vi "Send PING.vi"(8 "error in (no error)":errorcluster caption="entrée d'erreur (pas d'erreur)", 9 "timeout":i32=50, 10 "Frame Send":i32=10, 11 "@IP":string="192.168.0.100") -> (0 "error out":errorcluster caption="sortie d'erreur", 2 "Result/Request":bool[](array[boolean]), 3 "Result":bool)   [LabVIEW 2020, in "Library Commun.lvlib"]
uses:
  Library Commun.lvlib
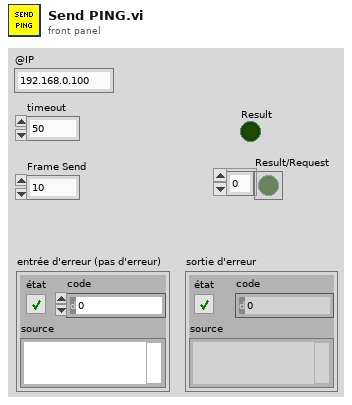
[diagram p1: front panel]
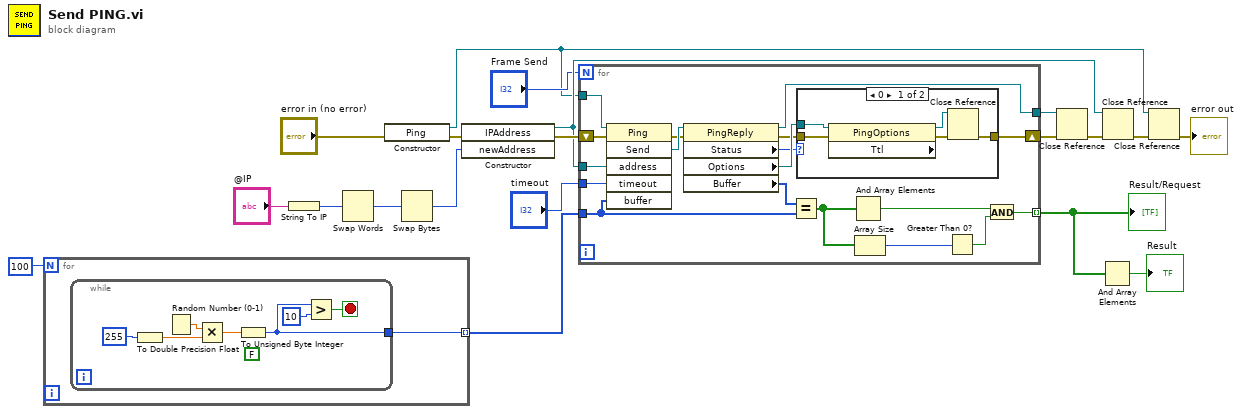
[diagram p0: block diagram]
diagram:
  n1 = for {
    N: 100 -> [_]
    tunnel: [w21] -> w9 mode=indexing
    n2 = while {
      tunnel: [w24] -> w21
      stop <- w22 stop-if-true
      (unwired) FALSE
      n3 = To Double Precision Float(number=u8 255 ("nombre")) -> (double precision float=w26:dbl)
      n4 = Random Number (0-1)() -> (number: 0 to 1=w27:dbl)
      n5 = Multiply(x=w27, y=w26) -> (x*y=w25:dbl)
      n6 = To Unsigned Byte Integer(number=w25) -> (unsigned 8bit integer=w24:u8)
      n7 = Greater?(x=w24, y=u8 10) -> (0:w22:bool)
    }
  }
  n8 = String To IP(1:"@IP") -> (0:w18:u32)
  n9 = Swap Words(1:w18) -> (0:w17:u32)
  n10 = constructor class="Ping"(error in="error in (no error)") -> (reference out=w1:refnum<k24>, error out=w20:errorcluster)  [unwired: 2 in, 1 out]
  n11 = Swap Bytes(anything=w17) -> (byte swapped=w16:u32)
  n12 = constructor class="IPAddress"(error in=w20, "newAddress"=w16) -> (reference out=w11:refnum<k24>, error out=w15:errorcluster)  [unwired: 2 in, 2 out]
  n13 = for {
    N: "Frame Send" -> [_]
    tunnel: w1 -> [w46]
    tunnel: "timeout" -> [w43]
    tunnel: [w41] -> w13
    tunnel: w11 -> [w40]
    tunnel: w9 -> [w37]
    tunnel: [w32] -> w6 mode=indexing
    shift-right: [w34] -> w8
    shift-left: w15 -> [w44]
    n14 = invoke class="Ping" method="Send"(reference=w46, error in=w44, "address"=w40, "timeout"=w43, "buffer"=w37) -> (error out=w42:errorcluster, "Send"=w45:refnum<k24>)  [unwired: 1 in, 4 out]
    n15 = property on="Nœud de propriété" class="PingReply"(reference=w45, error in=w42) -> (reference out=w41:refnum<k24>, error out=w36:errorcluster, "Status"=w35:i32, "Options"=w39:refnum<k24>, "Buffer"=w38:u8[])
    n16 = Equal?(x=w38, y=w37) -> (x = y?=w31:bool[])
    n17 = case shown="0" w35 {
      tunnel: w39 -> [w51 _]
      tunnel: w36 -> [w50 w52]
      tunnel: [w48 w52] -> w34
      frame 0 {
        n18 = property on="Nœud de propriété" class="PingOptions" props=["Ttl"](reference=w51, error in=w50) -> (reference out=w49:refnum<k24>, error out=w47:errorcluster)  [unwired: 1 out]
        n19 = Close Reference(reference=w49, error in (no error)=w47) -> (error out=w48:errorcluster)
      }
      frame Default {
      }
    }
    n20 = And Array Elements(Boolean array=w31) -> (logical AND=w33:bool)
    n21 = Array Size(array=w31) -> (size(s)=w30:i32)
    n22 = Greater Than 0?(x=w30) -> (x > 0?=w29:bool)
    n23 = And(x=w33, y=w29) -> (x .and. y?=w32:bool)
  }
  "Result/Request" <- w6
  n24 = Close Reference(reference=w13, error in (no error)=w8) -> (error out=w12:errorcluster)
  n25 = And Array Elements(Boolean array=w6) -> (logical AND=→"Result":bool)
  n26 = Close Reference(reference=w11, error in (no error)=w12) -> (error out=w3:errorcluster)
  n27 = Close Reference(reference=w1, error in (no error)=w3) -> (error out=→"error out":errorcluster)
